vi "GetReserveState.vi"(8 "error in (no error)":errorcluster, 11 "SMO":refnum<class "SMO.lvclass">) -> (0 "error out":errorcluster, 2 "Reserve State":T1, 3 "SMO out":refnum<class "SMO.lvclass">)   [LabVIEW 2019, in "SMO.lvclass"]
doc: "JKI State Machine Objects (SMO) 1.3.0.56\nJKI - JKI\nCopyright (c) 2017, JKI"
uses:
  SMO.lvclass
  Typedefs/Reserve State--Enum.ctl
  SMO.lvclass/SMO.ctl
panel:
  # "For instructions on how to use the JKI State Machine Objects, examples and video tutorials, visit:\nhttp://jki.net/state-machine-objects/\n\nJKI State Machine Objects™\nhttp://jki.net/state-machine-objects/\nCopyright (C) 2005-2015, JKI <info@jki.net>\nALL RIGHTS RESERVED"
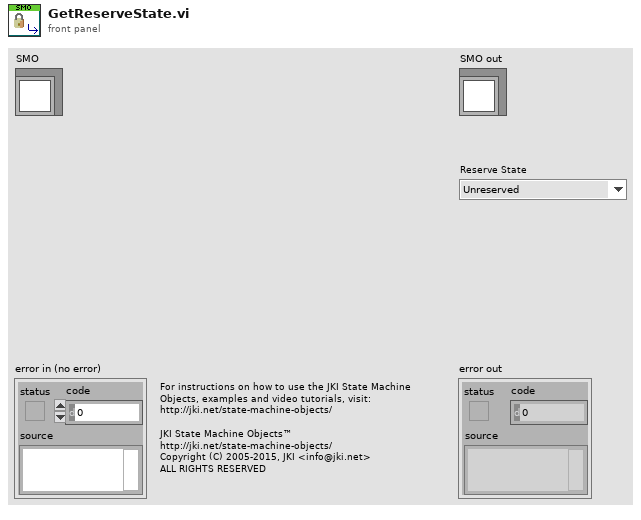
[diagram p1: front panel]
types:
  T1 = typedef "SMO.lvclass/Reserve State--Enum.ctl" = enum16{"Unreserved", "Reserved", "Self-locked"}
  T2 = typedef "SMO.lvclass/PrivateData--Ref.ctl" = refnum<data-value>
  T3 = typedef "SMO.lvclass/PrivateData--Cluster.ctl" = cluster{"Parent Call":T4, "Registered Processes":T5[], "Sync Notifier":refnum<notifier>, "Process Error Notifier":refnum<notifier>, "Protected Events":T6, "Public Events":T7, "SMO State":T8, "[Dependencies]":T9[], "[Attributes]":refnum<class "Attribute.lvclass">[], "Launcher Close":refnum<notifier>, "Caller Watchdog":refnum<queue>, "Accessibility":T10, "NbStaticDependencies":u32}
  T4 = typedef "SMO.lvclass/Parent Call--Enum.ctl" = enum16{"Allows parent to run", "Does not request parent to run"}
  T5 = typedef "SMO.lvclass/RegisteredProcessData--Cluster.ctl" = cluster{"Name":string, "Static VI Ref":refnum<vi>, "Running":bool, "NotifierRef":u32}
  T6 = typedef "SMO.lvclass/Protected Events.ctl" = cluster{"StopProcesses":refnum<user-event>, "AbortProcesses":refnum<user-event>, "Config Changed":refnum<user-event>, "Dependency":refnum<user-event>}
  T7 = typedef "SMO.lvclass/Public Events.ctl" = cluster{"Error":refnum<user-event>, "State":refnum<user-event>, "Reserve State":refnum<user-event>}
  T8 = typedef "SMO.lvclass/SMOState --Enum.ctl" = enum16{"unknown", "Created", "Started", "Stopped"}
  T9 = typedef "SMO.lvclass/SMO Dependency--Cluster.ctl" = cluster{"Dependency":refnum<class "SMO.lvclass">, "Level":string}
  T10 = typedef "SMO.lvclass/Accessibility--Cluster.ctl" = cluster{"Lock Key":string, "Reserve State":T1}
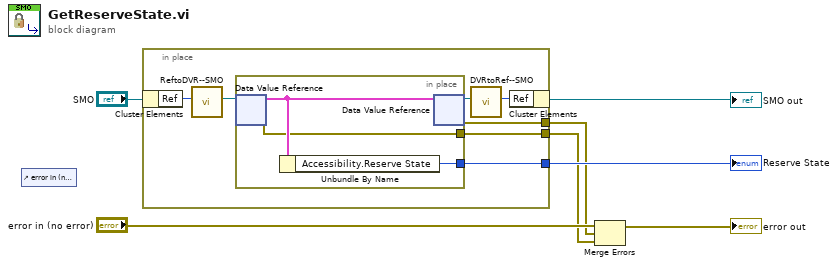
[diagram p0: block diagram]
diagram:
  n1 = control-ref of="error in (no error)"() -> ()  [unwired: 1 out]
  n2 = in-place {
    in-place-border: [w14] -> w3
    in-place-border: [w13] -> w1
    in-place-border: [w12] -> w2
    n3 = in-place-cluster #1("SMO") -> ("Ref"=w11:u32)
    n4 = call "ReftoDVR--SMO.vi"("Ref"=w11) -> ("Ref"=w10:T2)  [unwired: 10 in]
    n5 = in-place {
      in-place-border: [w17] -> w14
      in-place-border: [w15] -> w12
      n6 = in-place-dvr #2(w10) -> (w16:T3, w15:errorcluster)
      n7 = Unbundle By Name(w16) -> ("Accessibility.Reserve State"=w17:T1)
      n8 = in-place-dvr #2(w16) -> (w9:T2, w13:errorcluster)
    }
    n9 = call "DVRtoRef--SMO.vi"("Ref"=w9) -> ("Ref"=w8:u32)  [unwired: 10 in]
    n10 = in-place-cluster #1("Ref"=w8) -> (→"SMO out":refnum<class "SMO.lvclass">)
  }
  "Reserve State" <- w3
  n11 = Merge Errors("error in (no error)", w1, w2) -> (→"error out":errorcluster)
